vi "rutaUDLejecutable.vi"(5 "Database Path In":path) -> (2 "Database Path Out":path)   [LabVIEW 2018]
doc: "This VI is modifying the database path if executed during runtime."
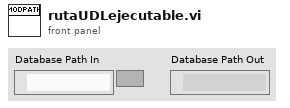
[diagram p1: front panel]
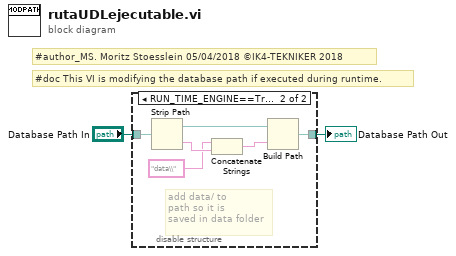
[diagram p0: block diagram]
diagram:
  # "#author_MS. Moritz Stoesslein 05/04/2018 ©IK4-TEKNIKER 2018"
  # "#doc This VI is modifying the database path if executed during runtime."
  n1 = disable-structure shown="RUN_TIME_ENGINE==True" {
    disable-tunnel: "Database Path In" -> [w3 w9]
    disable-tunnel: [w3 w8] -> w1
    frame condition #0 (active) {
      # "Do nothing"
    }
    frame condition #1 {
      # "add data/ to \npath so it is \nsaved in data folder"
      n2 = Strip Path(path=w9) -> (stripped path=w7:path, name=w5:string)
      n3 = Concatenate Strings("data\\" ("string"), w5) -> (w6:string)
      n4 = Build Path(base path=w7, name or relative path=w6) -> (appended path=w8:path)
    }
  }
  "Database Path Out" <- w1
